vi "LowSlope.vi"(1 "board":u32) -> ()   [LabVIEW 2015]
uses:
  ESLSCDLL.dll
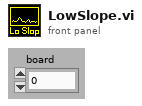
[diagram p1: front panel]
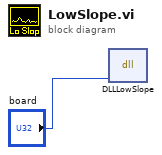
[diagram p0: block diagram]
diagram:
  n1 = dll-call lib="C:/ENTW/PCIE/64bit/lv64/lv64_labview2015/board.vis/ESLSCDLL.dll" fn="DLLLowSlope"("drv"="board") -> ()  [unwired: 5 in, 2 out]
